vi "PPMSDR_Archive.vi"   [LabVIEW 2013]
uses:
  <vilib>/lvdsc/NI_DSC.lvlib
types:
  T1 = cluster{"show status bar (T)":bool, "compact (T)":bool, "use * as wildcard (F)":bool}
  T2 = cluster{"show status bar (T)":bool, "compact (T)":bool, "use * as wildcard (F)":bool, "delete data from source database (F)":bool}
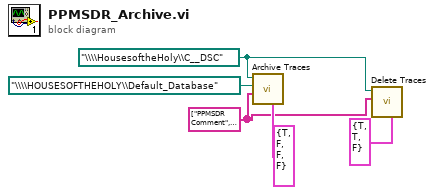
[diagram p0: block diagram]
diagram:
  w1 = string[] ["PPMSDR Comment", "PPMSDR Time Stamp (sec)", "PPMSDR Status (code)", "PPMSDR Temperature (K)", "PPMSDR Magnetic Field (Oe)", "PPMSDR Sample Position (deg)", "PPMSDR Bridge 1 Resistance (ohms)", "PPMSDR Bridge 1 Excitation (uA)", "PPMSDR Bridge 2 Resistance (ohms)", "PPMSDR Bridge 2 Excitation (uA)", "PPMSDR Bridge 3 Resistance (ohms)", "PPMSDR Bridge 3 Excitation (uA)", "PPMSDR Bridge 4 Resistance (ohms)", "PPMSDR Bridge 4 Excitation (uA)", "PPMSDR Signal 1 Vin (V)", "PPMSDR Signal 2 Vin (V)", "PPMSDR Digital Inputs (code)", "PPMSDR Drive 1 Iout (mA)", "PPMSDR Drive 1 Ipower (watts)", "PPMSDR Drive 2 Iout (mA)", "PPMSDR Drive 2 Ipower (watts)", "PPMSDR Pressure ()", "PPMSDR Map 20 ()", "PPMSDR Map 21 ()", "PPMSDR Map 22 ()", "PPMSDR Map 23 ()", "PPMSDR Map 24 ()", "PPMSDR Map 25 ()", "PPMSDR Map 26 ()", "PPMSDR Map 27 ()", "PPMSDR Map 28 ()", "PPMSDR Map 29 ()", "PPMSDR System Status (code)", "PPMSDR Setpoint (K)", "PPMSDR Magnet (Oe)", "PPMSDR Valve Position (deg)", "PPMSDR CIG Cernox (K)", "PPMSDR CIG Excit (uA)", "PPMSDR Plat Therm (K)", "PPMSDR Plat Excit (uA)", "PPMSDR Neck Therm (K)", "PPMSDR Neck Excit (uA)", "PPMSDR Spare Therm (K)", "PPMSDR Spare Excit (uA)", "PPMSDR Flow Rate (l min)", "PPMSDR Annulus Vacuum (V)", "PPMSDR Impedance (mode)", "PPMSDR Block Htr Cur (mA)", "PPMSDR Block Htr Pwr (W)", "PPMSDR Neck Htr Cur (mA)", "PPMSDR Neck Htr Pwr (W)", "PPMSDR Annulus Pres (Torr)", "PPMSDR System Pres (Torr)", "PPMSDR Tableless Map53 ()", "PPMSDR Tableless Map54 ()", "PPMSDR Redirected 55 ()", "PPMSDR Redirected 56 ()", "PPMSDR Redirected 57 ()", "PPMSDR Redirected 58 ()", "PPMSDR Redirected 59 ()", "PPMSDR EXT Flow (L min)", "PPMSDR Redirected 61 ()", "PPMSDR Seq Stat ()", "PPMSDR Sys Temp ()", "PPMSDR He Level ()", "PPMSDR Map 67 ()", "PPMSDR Map 68 ()", "PPMSDR Map 69 ()", "PPMSDR low res (A) read", "PPMSDR Hi res (A) read", "PPMSDR Mag (V) read", "PPMSDR Mag adj sc(I)set", "PPMSDR Sw heater state", "PPMSDR DAC  I  (cnts)", "PPMSDR Therm v", "PPMSDR KRPMs", "PPMSDR Pump temp (C)", "PPMSDR Pump power (W)", "PPMSDR High Vacuum mode", "PPMSDR Flapper state", "PPMSDR Regen htr flag", "PPMSDR iso flag", "PPMSDR BlockHeater(Ohm)", "PPMSDR NeckHeater(Ohm)", "PPMSDR Last 2 eng st", "PPMSDR Hires enable", "PPMSDR Mag (V) set", "PPMSDR Map 89 ()", "PPMSDR Map 90 ()", "PPMSDR Map 91 ()", "PPMSDR Map 92 ()", "PPMSDR Map 93 ()", "PPMSDR MAP 1", "PPMSDR MAP 2", "PPMSDR MAP 3", "PPMSDR MAP 4", "PPMSDR MAP 5", "PPMSDR MAP 6", "PPMSDR MAP 7", "PPMSDR MAP 8", "PPMSDR MAP 9", "PPMSDR MAP 10", "PPMSDR MAP 11", "PPMSDR MAP 12", "PPMSDR MAP 13", "PPMSDR MAP 14", "PPMSDR MAP 15", "PPMSDR MAP 16", "PPMSDR MAP 17", "PPMSDR MAP 18", "PPMSDR MAP 19", "PPMSDR MAP 20", "PPMSDR MAP 21", "PPMSDR MAP 22", "PPMSDR MAP 23", "PPMSDR MAP 24", "PPMSDR MAP 25", "PPMSDR MAP 26", "PPMSDR MAP 27", "PPMSDR MAP 28", "PPMSDR MAP 29", "PPMSDR MAP 30"] ("Array")
  w3 = path "\\\\HousesoftheHoly\\C__DSC" ("source database URL")
  n1 = call <vilib>:"Archive Traces.vi"("options"=T2 {"show status bar (T)"=TRUE, "compact (T)"=FALSE, "use * as wildcard (F)"=FALSE, "delete data from source database (F)"=FALSE}, "trace names"=w1, "destination database URL"=path "\\\\HOUSESOFTHEHOLY\\Default_Database", "source database URL"=w3) -> ()  [unwired: 5 in, 3 out]
  n2 = call <vilib>:"Delete Traces.vi"("options"=T1 {"show status bar (T)"=TRUE, "compact (T)"=TRUE, "use * as wildcard (F)"=FALSE}, "trace names"=w1, "database name"=w3) -> ()  [unwired: 7 in, 2 out]
